vi "例2.2求平均数.vi"(1 "B":dbl, 2 "A":dbl) -> (0 "Result":dbl)   [LabVIEW 2012]
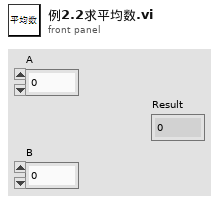
[diagram p1: front panel]
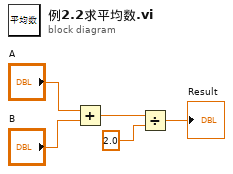
[diagram p0: block diagram]
diagram:
  n1 = Add(x="A", y="B") -> (x+y=w3:dbl)
  n2 = Divide(x=w3, y=2.0) -> (x/y=→"Result":dbl)
